vi "Send command.vi"(7 "error in":errorcluster, 9 "MES url":string="https://eur05.safelinks.protection.outlook.com/?url=http%3A%2F%2F10.186.160.170%2FNidecMES_DataLinkage_Api%2FWebService%2FContactAndRegisterWithNmaSapService.asmx&data=05%7C02%7Cmilica.bokcic%40noffz.com%7C5dac078428e14667fedf08de39595599%7C2e83dfe143ac4a97b8dc1c3165e7dc35%7C1%7C0%7C639011253504459186%7CUnknown%7CTWFpbGZsb3d8eyJFbXB0eU1hcGkiOnRydWUsIlYiOiIwLjAuMDAwMCIsIlAiOiJXaW4zMiIsIkFOIjoiTWFpbCIsIldUIjoyfQ%3D%3D%7C0%7C%7C%7C&sdata=ZY%2FOyToJH5s9%2F4dphrEPgMy%2BejIHhfaNk%2B7PkGqYvSo%3D&reserved=0", 10 "MES Request":string) -> (0 "error out":errorcluster, 3 "MES Response":string)   [LabVIEW 2023, in "MES.lvlib"]
uses:
  MES.lvlib
  <vilib>/httpClient/LabVIEWHTTPClient.lvlib
  <vilib>/httpClient/PUTBuffer.vi
  <vilib>/httpClient/POSTBuffer.vi
panel:
  in  "Boolean":bool=TRUE
  out "headers":string
  out "body":string
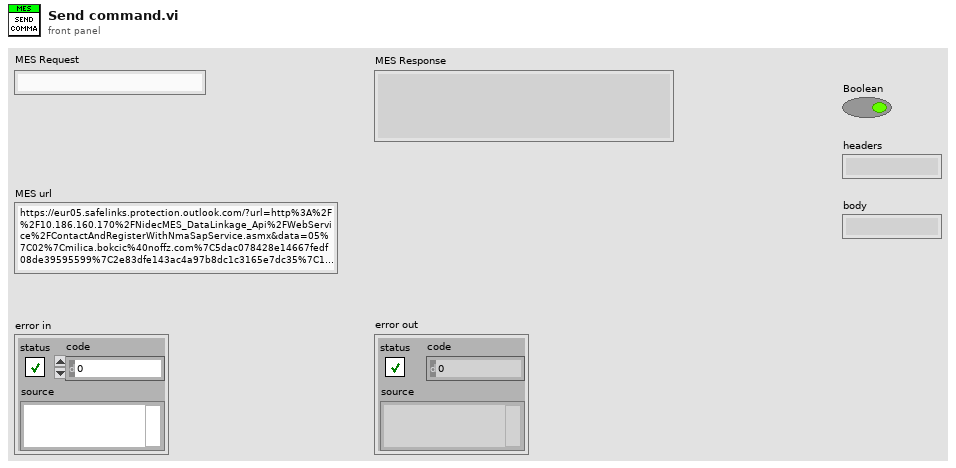
[diagram p1: front panel]
types:
  T1 = typedef "LabVIEWHTTPClient.lvlib/ClientHandle.ctl" = refnum<k1>
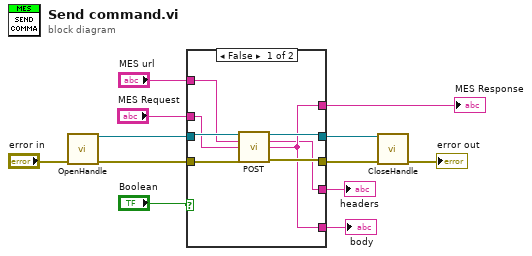
[diagram p0: block diagram]
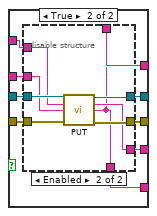
[diagram p2: hidden frame]
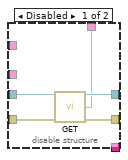
[diagram p3: hidden frame]
diagram:
  n1 = call <vilib>:"OpenHandle.vi"("error in (no error)"="error in") -> ("client handle out"=w12:T1, "error out"=w8:errorcluster)  [unwired: 13 in]
  n2 = case shown="False" "Boolean" {
    tunnel: w12 -> [w18 w29]
    tunnel: [w17 w28] -> w11
    tunnel: [w19 w27] -> w10
    tunnel: w8 -> [w20 w26]
    tunnel: [w16 w25] -> w6
    tunnel: "MES url" -> [w14 w24]
    tunnel: "MES Request" -> [w13 w23]
    tunnel: [w16 w22] -> w3
    tunnel: [w15 w21] -> w2
    frame False {
      n3 = call-poly <vilib>:"POST.vi"("client handle"=w18, "url"=w14, "buffer"=w13, "error in (no error)"=w20) -> ("client handle out"=w17:T1, "headers"=w15:string, "body"=w16:string, "error out"=w19:errorcluster)  [unwired: 8 in]
    }
    frame True {
      n4 = disable-structure shown="Enabled" {
        disable-tunnel: w29 -> [w34 w42]
        disable-tunnel: [w33 w41] -> w28
        disable-tunnel: [w32 w37] -> w27
        disable-tunnel: w26 -> [w31 w38]
        disable-tunnel: [w30 w35] -> w25
        disable-tunnel: w24 -> [_ w40]
        disable-tunnel: w23 -> [_ w39]
        disable-tunnel: [_ w35] -> w22
        disable-tunnel: [_ w36] -> w21
        frame Disabled {
          n5 = call <vilib>:"GET.vi"("client handle"=w34, "error in (no error)"=w31) -> ("client handle out"=w33:T1, "body"=w30:string, "error out"=w32:errorcluster)  [unwired: 10 in, 1 out]
        }
        frame Enabled {
          n6 = call-poly <vilib>:"PUT.vi"("client handle"=w42, "url"=w40, "buffer"=w39, "error in (no error)"=w38) -> ("client handle out"=w41:T1, "headers"=w36:string, "body"=w35:string, "error out"=w37:errorcluster)  [unwired: 8 in]
        }
      }
    }
  }
  "MES Response" <- w6
  "body" <- w3
  "headers" <- w2
  n7 = call <vilib>:"CloseHandle.vi"("client handle"=w11, "error in (no error)"=w10) -> ("error out"=→"error out":errorcluster)  [unwired: 13 in]
